vi "sub_map-providers_check.vi"() -> ()   [LabVIEW 2019]
uses:
  C:/Users/WeGo/Documents/GitHub/Ycar/LabVIEW/Gmap/dll/GMap.NET.Core.dll
  dll/GMap.NET.Core.dll
panel:
  out "에러 출력":errorcluster
  in  "Ring menu":u16(ring) items=["ArcGIS_DarbAE_Q2_2011_NAVTQ_Eng_V5_MapProvider", "ArcGIS_Imagery_World_2D_Map", "ArcGIS_ShadedRelief_World_2D_Map", "ArcGIS_StreetMap_World_2D_Map", "ArcGIS_Topo_US_2D_Map", "ArcGIS_World_Physical_Map", "ArcGIS_World_Shaded_Relief_Map", "ArcGIS_World_Street_Map", "ArcGIS_World_Terrain_Base_Map", "ArcGIS_World_Topo_Map", "BingHybridMap", "BingMap", "BingSatelliteMap", "CloudMade, Demo", "CzechHistoryMap", "CzechHybridMap", "CzechMap", "CzechSatelliteMap", "CzechTuristMap", "GoogleChinaHybridMap", "GoogleChinaMap", "GoogleChinaSatelliteMap", "GoogleChinaTerrainMap", "GoogleHybridMap", "GoogleKoreaHybridMap", "GoogleKoreaMap", "GoogleKoreaSatelliteMap", "GoogleMap", "GoogleSatelliteMap", "GoogleTerrainMap", "LatviaMap", "Lithuania 2.5d Map", "LithuaniaHybridMapOld", "LithuaniaHybridMap", "LithuaniaMap", "LithuaniaOrtoFotoMapOld", "LithuaniaOrtoFotoMap", "LithuaniaTOP50", "MapBender, WMS demo", "NearHybridMap", "NearMap", "NearSatelliteMap", "None", "OpenCycleLandscapeMap", "OpenCycleMap", "OpenCycleTransportMap", "OpenSeaMapHybrid", "OpenStreet4UMap", "OpenStreetMapQuestHybrid", "OpenStreetMapQuestSattelite", "OpenStreetMapQuest", "OpenStreetMap", "OviHybridMap", "OviMap", "OviSatelliteMap", "OviTerrainMap", "SpainMap", "TurkeyMap", "WikiMapiaMap", "YahooHybridMap", "YahooMap", "YahooSatelliteMap", "YandexHybridMap", "YandexMap", "YandexSatelliteMap"]
  in  "콤보 박스":string(combo)
  out "IdxInitPrvd":string
  out "SelProvider":refnum<k24>
  in  "InitProviders":string caption="ReqProvider"
  out "arr1DProviders":string[](array[string])
  out "arrRefProviders":refnum<k24>[](array[refnum])
  out "cmbProviders":cluster{"Name":string, string}[](array[cluster])
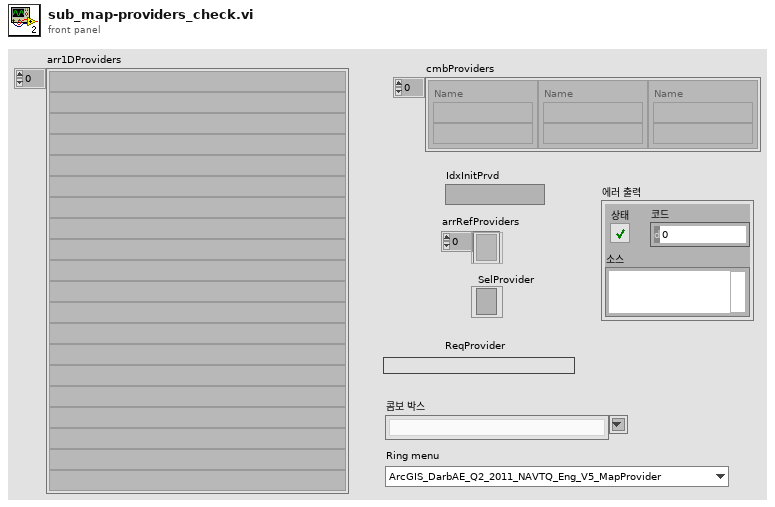
[diagram p1: front panel]
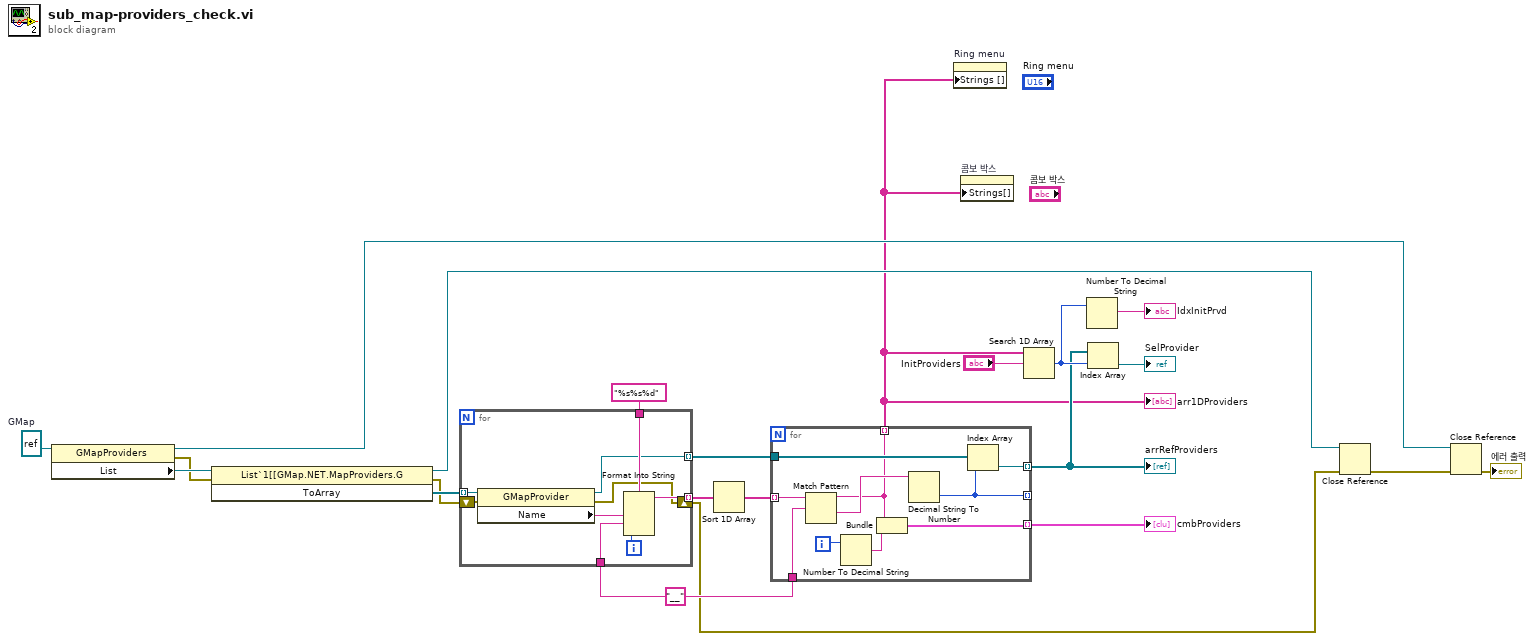
[diagram p0: block diagram]
diagram:
  w16 = "__" ("regular expression")
  w9 = refnum<k24> refnum  # GMap
  n1 = property class="GMapProviders"(reference=w9) -> (reference out=w7:refnum<k24>, error out=w5:errorcluster, "List"=w20:refnum<k24>)  [unwired: 1 in]
  n2 = invoke class="List`1[[GMap.NET.MapProviders.G" method="ToArray"(reference=w20, error in=w5) -> (reference out=w8:refnum<k24>, error out=w3:errorcluster, "ToArray"=w21:refnum<k24>[])  [unwired: 1 in]
  n3 = for {
    tunnel: w21 -> [w30] mode=indexing
    tunnel: [w31] -> w18 mode=indexing
    tunnel: [w24] -> w19 mode=indexing
    tunnel: "%s%s%d" ("format string") -> [w28]
    tunnel: w16 -> [w26]
    shift-right: [w23] -> w2
    shift-left: w3 -> [w25]
    i -> [w27]
    n4 = property class="GMapProvider"(reference=w30, error in=w25) -> (reference out=w24:refnum<k24>, error out=w23:errorcluster, "Name"=w29:string)
    n5 = Format Into String(format string=w28, w29, w26, w27) -> (resulting string=w31:string)  [unwired: 2 in, 1 out]
  }
  n6 = Sort 1D Array(array=w18) -> (sorted array=w15:string[])
  n7 = for {
    tunnel: w15 -> [w38] mode=indexing
    tunnel: [w39] -> w22 mode=indexing
    tunnel: w19 -> [w36]
    tunnel: [w35] -> w12 mode=indexing
    tunnel: w16 -> [w34]
    tunnel: [w33] -> w4 mode=indexing
    tunnel: [w32] -> _ mode=indexing
    i -> [w40]
    n8 = Match Pattern(string=w38, regular expression=w34) -> (before substring=w33:string, after substring=w37:string)  [unwired: 1 in, 2 out]
    n9 = Number To Decimal String(number=w40) -> (decimal integer string=w41:string)  [unwired: 1 in]
    n10 = Bundle(w33, w41) -> (w39:cluster{string, string})  [unwired: 1 in]
    n11 = Decimal String To Number(string=w37) -> (number=w32:i32)  [unwired: 2 in, 1 out]
    n12 = Index Array(array=w36, index=w32) -> (element=w35:refnum<k24>)
  }
  "cmbProviders" <- w22
  "arrRefProviders" <- w12
  "arr1DProviders" <- w4
  n13 = property on="Ring menu" class="Ring (엄격한)"("Strings []"=w4) -> ()  [unwired: 2 in, 2 out]
  n14 = property on="콤보 박스" class="CmbBox"("Strings[]"=w4) -> ()  [unwired: 2 in, 2 out]
  n15 = Search 1D Array(1D array=w4, element="InitProviders") -> (index of element=w13:i32)  [unwired: 1 in]
  n16 = Number To Decimal String(number=w13) -> (decimal integer string=→"IdxInitPrvd":string)  [unwired: 1 in]
  n17 = Index Array(array=w12, index=w13) -> (element=→"SelProvider":refnum<k24>)
  n18 = Close Reference(reference=w8, error in (no error)=w2) -> (error out=w6:errorcluster)
  n19 = Close Reference(reference=w7, error in (no error)=w6) -> (error out=→"에러 출력":errorcluster)
